vi "SetPeakCurrent.vi"(0 "handle in":i32, 1 "UnitAddress (0)":u16, 2 "MotNr (0+1)":enum8{"0+1", "2+3", "4+5"}(ring), 5 "error in(no error)":errorcluster, 9 "Imax (50%)":T1=50.0 min=0.0 max=100.0) -> (14 "handle out":i32, 19 "error out":errorcluster)   [LabVIEW 2014, in "Sixpack - Driver.lvlib"]
doc: "CMD $10\nBefehl legt den Maximalstrom der jeweiligen Achse fest. Der Wert gilt für jeweils zwei Motoren."
uses:
  Sixpack - Driver.lvlib
  PeakCurrent.ctl
  DLL/PackDLL.dll
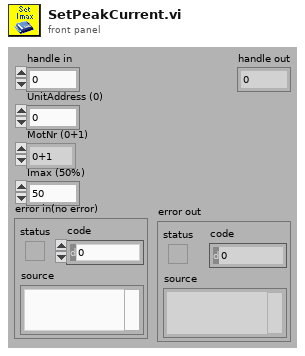
[diagram p1: front panel]
types:
  T1 = typedef "Sixpack - Driver.lvlib/PeakCurrent.ctl" = dbl
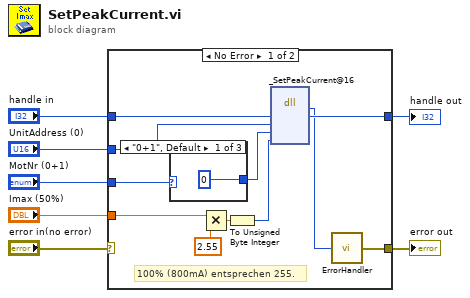
[diagram p0: block diagram]
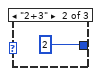
[diagram p2: hidden frame]
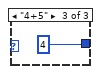
[diagram p3: hidden frame]
diagram:
  n1 = case shown="No Error" "error in(no error)" {
    selector: "error in(no error)" -> [_ w23]
    tunnel: "handle in" -> [w18 w22]
    tunnel: [w17 w22] -> w6
    tunnel: "UnitAddress (0)" -> [w16 _]
    tunnel: "MotNr (0+1)" -> [w15 _]
    tunnel: "Imax (50%)" -> [w9 _]
    tunnel: [w10 w23] -> w2
    frame No Error {
      # "100% (800mA) entsprechen 255."
      n2 = case shown="\"0+1\", Default" w15 {
        tunnel: [u8 0 ("MotNr") u8 2 ("MotNr") u8 4 ("MotNr")] -> w14
        frame "0+1", Default {
        }
        frame "2+3" {
        }
        frame "4+5" {
        }
      }
      n3 = Multiply(x=w9, y=2.55) -> (x*y=w8:T1)
      n4 = To Unsigned Byte Integer(number=w8) -> (unsigned 8bit integer=w13:u8)
      n5 = dll-call lib="D:/CS-Source/LV2014/GPL/instr.lib/SixPack/PackDLL/DLL/PackDLL.dll" fn="_SetPeakCurrent@16" label="SetPeakCurrent"("HANDLE"=w18, "UnitAddress"=w16, "MotNr"=w14, "Imax"=w13) -> ("BOOLEAN"=w11:i8, "HANDLE"=w17:i32)  [unwired: 6 in, 2 out]
      n6 = call "ErrorHandler.vi"("BOOLEAN"=w11) -> ("error out"=w10:errorcluster)
    }
    frame Error {
    }
  }
  "handle out" <- w6
  "error out" <- w2
